vi "Sub_Dial2.vi"() -> (0 "OUT":i32)   [LabVIEW 2019]
panel:
  in  "Cluster":T1
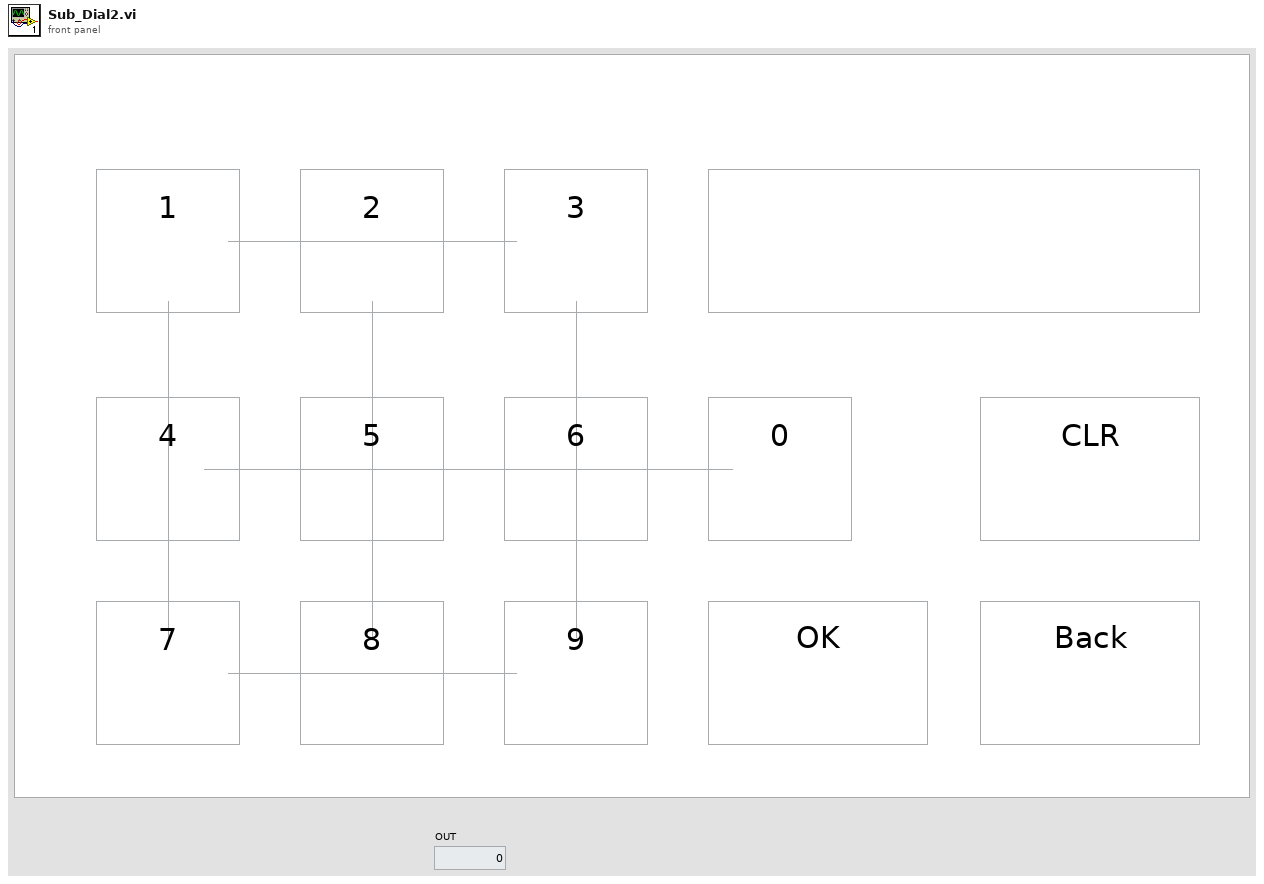
[diagram p1: front panel]
types:
  T1 = cluster{"1":bool, "2":bool, "3":bool, "4":bool, "5":bool, "6":bool, "7":bool, "8":bool, "9":bool, "STOP":bool, "0":bool, "String":string, "CLR":bool, "BACK":bool}
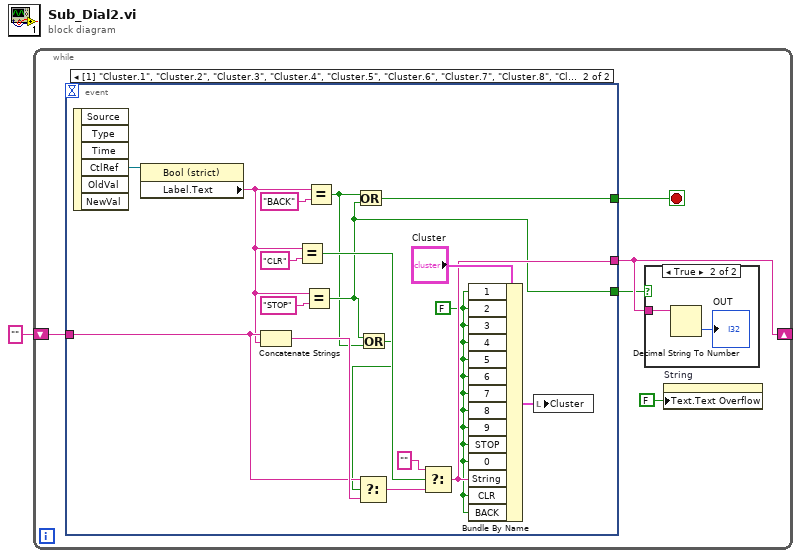
[diagram p0: block diagram]
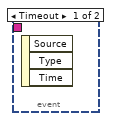
[diagram p3: hidden frame]
diagram:
  n1 = while {
    shift-right: [w4] -> _
    shift-left: "" -> [w6]
    stop <- w5 stop-if-true
    n2 = event shown="[1] \"Cluster.1\", \"Cluster.2\", \"Cluster.3\", \"Cluster.4\", \"Cluster.5\", \"Cluster.6\", \"Cluster.7\", \"Cluster.8\", \"Cluster.9\", \"Cluster.0\", \"Cluster.STOP\", \"Cluster.CLR\", \"Cluster.BACK\": Value Change" {
      selector: _ -> [_ _]
      dyn-events: _ -> [_ _]
      timeout: _ -> [_ _]
      tunnel: [_ w13] -> w5
      tunnel: w6 -> [_ w16]
      tunnel: [_ w19] -> w4
      tunnel: [_ w11] -> w3
      event Timeout {
        n3 = event-data() -> ()  [unwired: 1 in, 3 out]
      }
      event "Cluster.1", "Cluster.2", "Cluster.3", "Cluster.4", "Cluster.5", "Cluster.6", "Cluster.7", "Cluster.8", "Cluster.9", "Cluster.0", "Cluster.STOP", "Cluster.CLR", "Cluster.BACK": Value Change {
        w12 = FALSE
        n4 = event-data() -> ("CtlRef"=w26:refnum<vi>)  [unwired: 1 in, 5 out]
        n5 = property class="Bool (strict)"(reference=w26) -> ("Label.Text"=w15:string)  [unwired: 1 in, 2 out]
        n6 = Concatenate Strings(w16, w15) -> (w17:string)
        n7 = Equal?(x=w15, y="CLR") -> (x = y?=w21:bool)
        n8 = Equal?(x=w15, y="STOP") -> (x = y?=w11:bool)
        n9 = Equal?(x=w15, y="BACK") -> (x = y?=w10:bool)
        n10 = Or(x=w10, y=w11) -> (x .or. y?=w13:bool)
        n11 = Or(x=w11, y=w10) -> (x .or. y?=w9:bool)
        n12 = Select(t=w16, s=w9, f=w17) -> (s? t:f=w18:string)
        n13 = Select(t="", s=w21, f=w18) -> (s? t:f=w19:string)
        n14 = Bundle By Name(cluster="Cluster", "1"=w12, "2"=w12, "3"=w12, "4"=w12, "5"=w12, "6"=w12, "7"=w12, "8"=w12, "9"=w12, "STOP"=w12, "0"=w12, "String"=w19, "CLR"=w12, "BACK"=w12) -> (w23:T1)
        n15 = local write "Cluster"(w23) -> ()
      }
    }
    n16 = case shown="True" w3 {
      tunnel: w4 -> [_ w8]
      frame False {
      }
      frame True {
        n17 = Decimal String To Number(string=w8) -> (number=→"OUT":i32)  [unwired: 2 in, 1 out]
      }
    }
    n18 = property on="String" class="Str"("Text.Text Overflow"=FALSE) -> ()  [unwired: 2 in, 2 out]
  }
